vi "SDG60SelectChannel.vi"(2 "error in (no error)":errorcluster, 4 "Channel (1: Channel1)":u16(ring)=1 items=["Channel1"=1, "Channel2"=2], 5 "VISA resource name":refnum<visa-resource-name>="USB0::0xF4EC::0x1101::SDG6XEBC5R0119::INSTR") -> (0 "error out":errorcluster, 1 "VISA resource name out":refnum<visa-resource-name>)   [LabVIEW 2018]
doc: "Configures the output impedance and source impedance for the channel you specify."
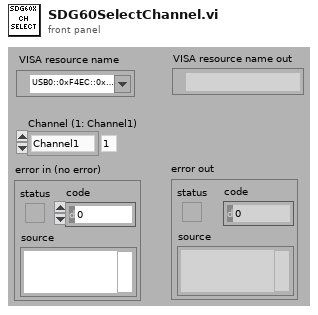
[diagram p1: front panel]
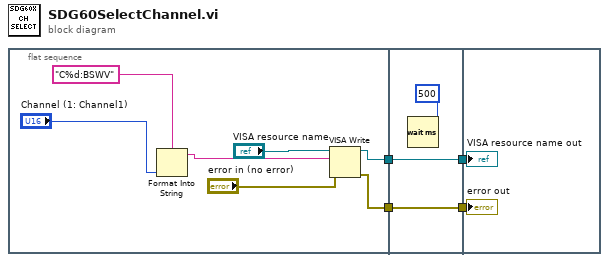
[diagram p0: block diagram]
diagram:
  n1 = flat-sequence {
    tunnel: [w6] -> w4
    tunnel: [w5] -> w2
    tunnel: w4 -> [w14]
    tunnel: [w14] -> w3
    tunnel: w2 -> [w13]
    tunnel: [w13] -> w1
    tunnel: w3 -> [w16]
    tunnel: w1 -> [w15]
    frame #0 {
      n2 = Format Into String(format string="C%d:BSWV", "Channel (1: Channel1)") -> (resulting string=w7:string)  [unwired: 2 in, 1 out]
      n3 = VISA Write(VISA resource name="VISA resource name", write buffer=w7, error in (no error)="error in (no error)") -> (VISA resource name out=w6:refnum<visa-resource-name>, error out=w5:errorcluster)  [unwired: 1 out]
    }
    frame #1 {
      n4 = Wait (ms)(milliseconds to wait=500) -> ()  [unwired: 1 out]
    }
    frame #2 {
      "error out" <- w15
      "VISA resource name out" <- w16
    }
  }
